vi "EMV Detect Flow Stop.vi"(0 ".NET Refnum in":refnum<k24>, 1 "Mixing Valve.MixValveAbsoluteStepPosition (0x400B)":i16, 2 "Mixing Valve.Flow State (0x4009)":u8, 5 "T7 History Input":dbl[](array[numeric]), 11 "error in (no error)":errorcluster, 13 "Abnormal Input Temperature":dbl=90.0) -> (4 "GEA2 Reference Out":refnum<k24>, 6 "Current T7 Temperatures Output":dbl[](array[numeric]), 8 "End of Flow Detection?":bool, 15 "error out":errorcluster)   [LabVIEW 2016]
uses:
  C:/TechnologyLab/NI-2010/Drivers/GEA3 Toolkit/GEA3 DLL Source/GeaCommunication.dll
  Drivers/GEA3 Toolkit/GEA3 DLL Source/GeaCommunication.dll
panel:
  in  "T7_DELTA_INDICATING_FLOW":dbl
  in  "Cold Water Supply Temperature":dbl
  in  "Detection Slope":dbl=0.2 format="%#_13g"
  in  "T7 STOP-T6 FLOW -THRESHOLD":dbl
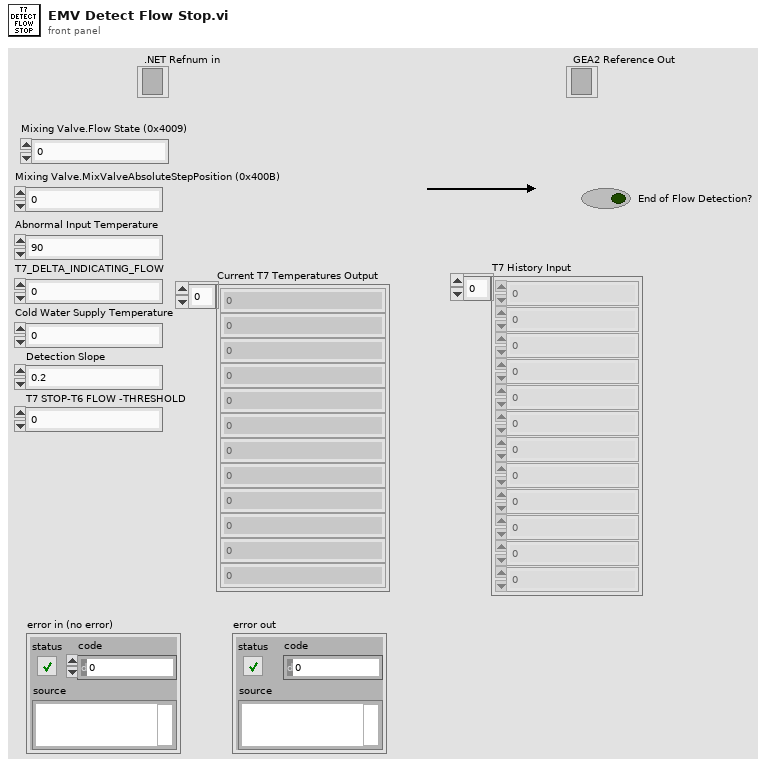
[diagram p1: front panel]
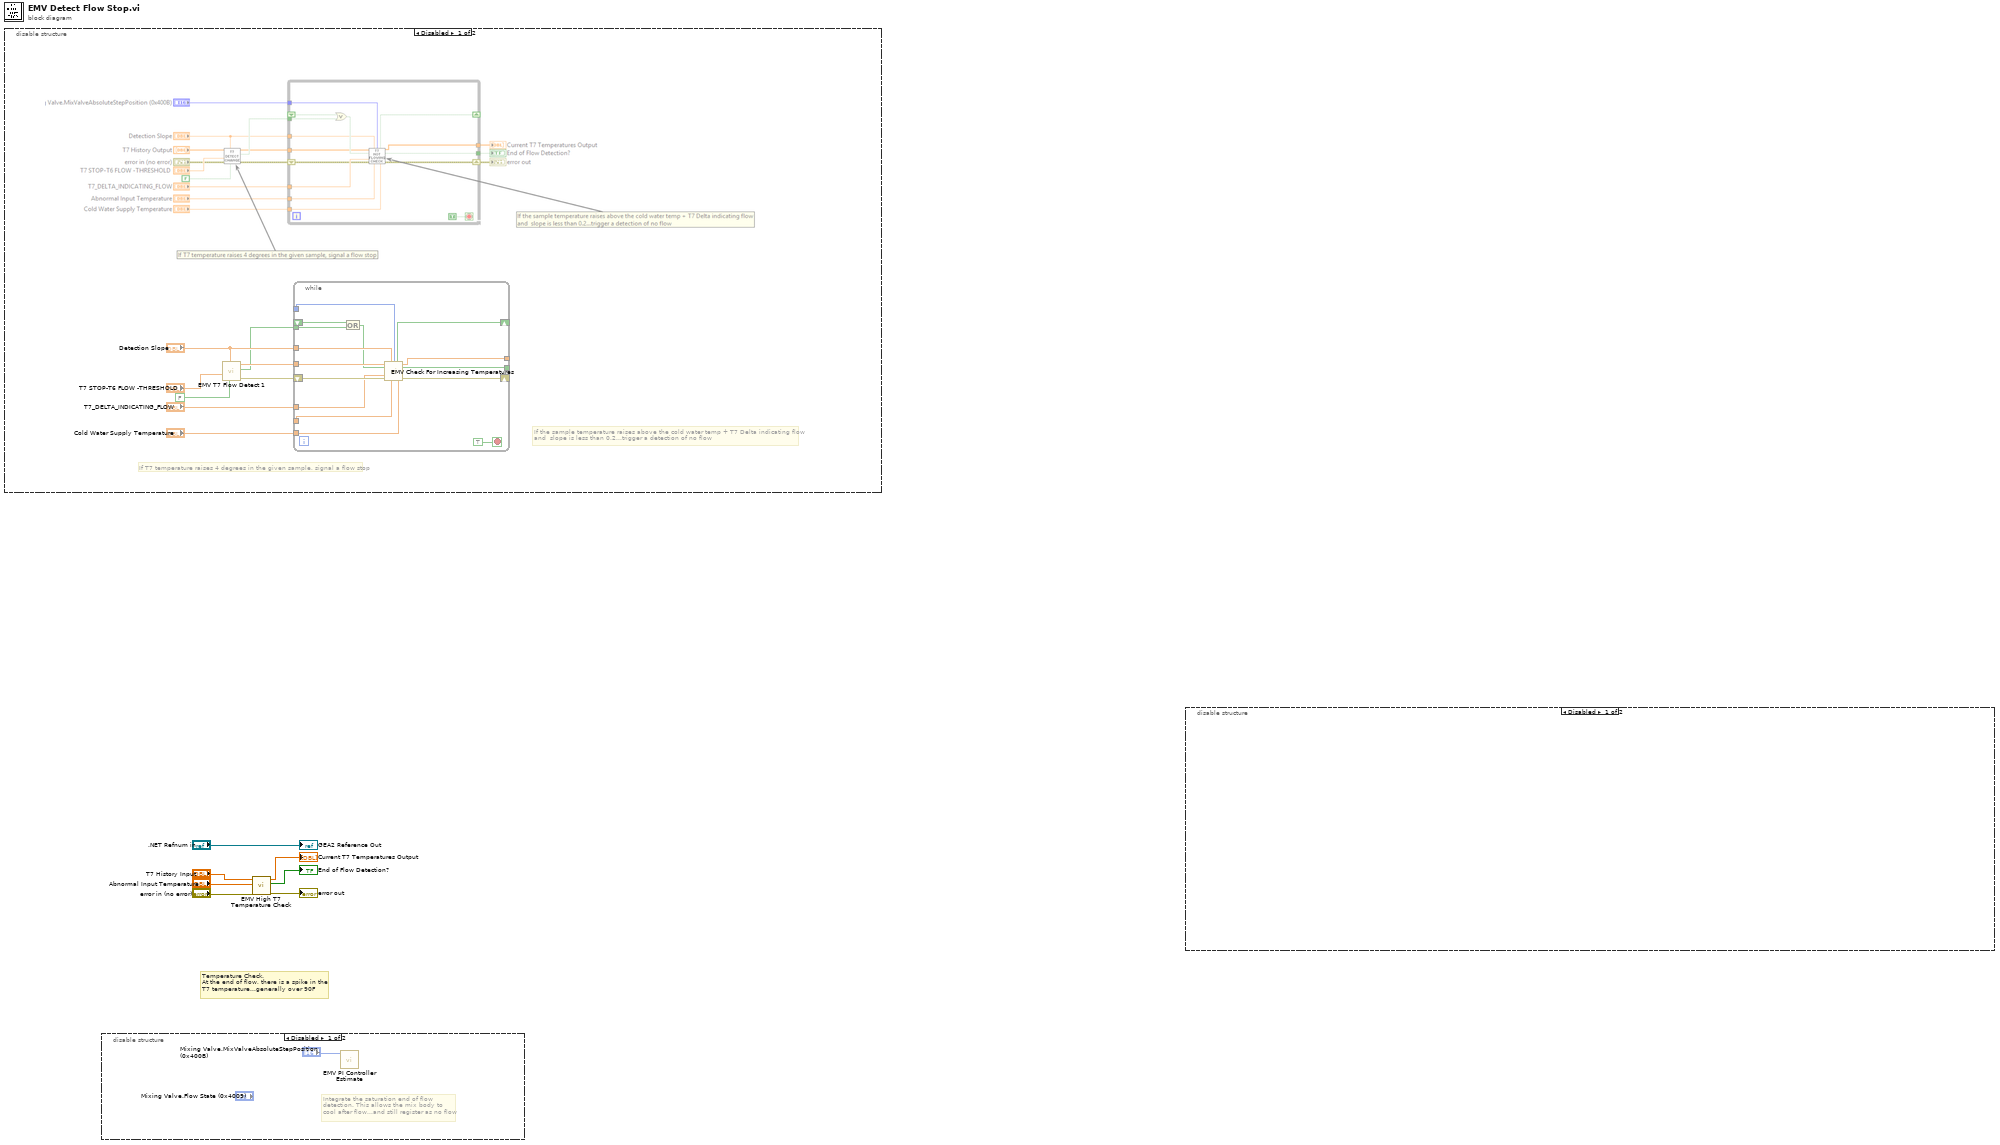
[diagram p0: block diagram]
diagram:
  # "Temperature Check.\nAt the end of flow, there is a spike in the \nT7 temperature...generally over 90F"
  n1 = disable-structure shown="Disabled" {
    frame Disabled {
      # "If the sample temperature raises above the cold water temp + T7 Delta indicating flow\nand  slope is less than 0.2...trigger a detection of no flow"
      # "If T7 temperature raises 4 degrees in the given sample, signal a flow stop"
      n2 = call "EMV T7 Flow Detect 1.vi"("Detect Flow Start?"=FALSE, "Detection Slope"="Detection Slope", "T7_DELTA_FLOW_THRESHOLD"="T7 STOP-T6 FLOW -THRESHOLD") -> ("error out"=w12:errorcluster, "Detection?"=w8:bool, "Current T7 Temperatures Output"=w9:dbl[])  [unwired: 5 in, 1 out]
      n3 = while {
        tunnel: "Cold Water Supply Temperature" -> [w30]
        tunnel: "T7_DELTA_INDICATING_FLOW" -> [w20]
        tunnel: [w27] -> _
        tunnel: "Detection Slope" -> [w26]
        tunnel: w9 -> [w25]
        shift-right: [w29] -> _
        shift-left: w12 -> [w28]
        shift-right: [w23] -> _
        shift-left: _ -> [w22]
        tunnel: w8 -> [w21]
        tunnel: _ -> [w18]
        tunnel: _ -> [w17]
        tunnel: [w16] -> _
        stop <- TRUE stop-if-true
        n4 = Or(x=w22, y=w21) -> (x .or. y?=w19:bool)
        n5 = call "EMV Check For Increasing Temperatures.vi"("Current T7 Temperatures"=w25, "Detection Slope"=w26, "Mixing Valve.MixValveAbsoluteStepPosition (0x400B)"=w17, "T7 Detection?"=w19, "T7_DELTA_INDICATING_FLOW"=w20, "error in (no error)"=w28, "Abnormal Input Temperature"=w18, "Cold Water Supply Temperature"=w30) -> ("Trigger Lock"=w23:bool, "Current T7 Temperatures Output"=w27:dbl[], "End of Flow Detection?"=w16:bool, "error out"=w29:errorcluster)  [unwired: 4 in]
      }
    }
    frame Enabled {
    }
  }
  n6 = disable-structure shown="Disabled" {
    frame Disabled {
      # "Integrate the saturation end of flow\ndetection. This allows the mix body to \ncool after flow...and still register as no flow"
      n7 = call "EMV PI Controller Estimate.vi"("Mixing Valve.MixValveAbsoluteStepPosition (0x400B)"="Mixing Valve.MixValveAbsoluteStepPosition (0x400B)") -> ()  [unwired: 9 in, 2 out]
    }
    frame Enabled {
    }
  }
  n8 = call "EMV High T7 Temperature Check.vi"("error in (no error)"="error in (no error)", "Abnormal Input Temperature"="Abnormal Input Temperature", "T7 History"="T7 History Input") -> ("error out"=→"error out":errorcluster, "Hot Inlet Water?"=→"End of Flow Detection?":bool, "T6 History Output"=→"Current T7 Temperatures Output":dbl[])  [unwired: 6 in]
  n9 = disable-structure shown="Disabled" {
    frame Disabled {
    }
    frame Enabled {
    }
  }
  "GEA2 Reference Out" <- ".NET Refnum in"
